vi "Read_data.vi"(0 "DVR in":refnum<data-value>, 5 "Type":string, 11 "error in (no error)":errorcluster) -> (4 "DVR Out":refnum<data-value>, 6 "DATA":T1, 15 "error out":errorcluster)   [LabVIEW 2020, in "With Data.lvclass"]
doc: "Read data to notifier."
uses:
  Classes/Children/Intra-Application/Children/With Data/With Data.lvclass
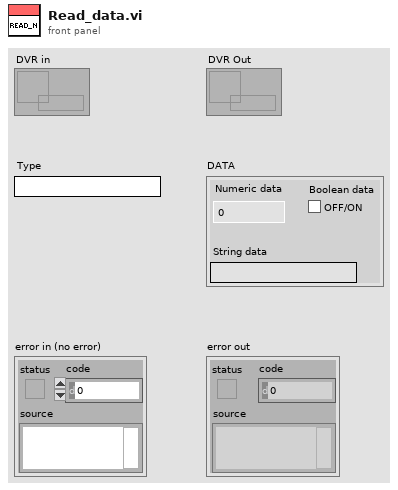
[diagram p1: front panel]
types:
  T1 = cluster{"Numeric data":dbl, "String data":string, "Boolean data":bool}
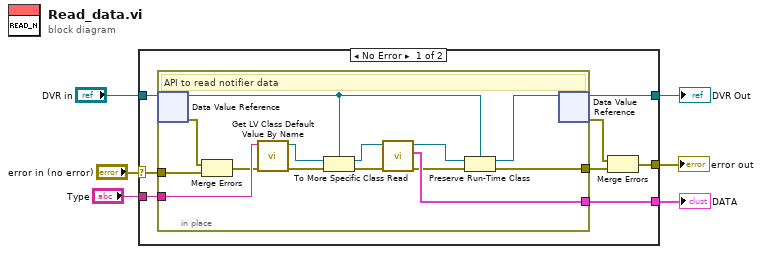
[diagram p0: block diagram]
diagram:
  n1 = case shown="No Error" "error in (no error)" {
    selector: "error in (no error)" -> [w14 w30]
    tunnel: [w11 w30] -> w5
    tunnel: [w10 _] -> w4
    tunnel: "DVR in" -> [w9 w29]
    tunnel: [w8 w29] -> w1
    tunnel: "Type" -> [w7 _]
    frame No Error {
      n2 = in-place "In Place Element Structure" {
        in-place-border: [w18] -> w13
        in-place-border: w14 -> [w27]
        in-place-border: [w20] -> w10
        in-place-border: w7 -> [w22]
        # "API to read notifier data"
        n3 = in-place-dvr #1(w9) -> (w16:refnum<class "With Data.lvclass">, w28:errorcluster)
        n4 = Merge Errors(w28, w27) -> (w21:errorcluster)
        n5 = call <vilib>:"Get LV Class Default Value By Name.vi"("error in (no error)"=w21, "class name"=w22) -> ("error out"=w23:errorcluster, "object"=w25:refnum<class>)  [unwired: 8 in]
        n6 = To More Specific Class(target class=w16, reference=w25, error in=w23) -> (specific class reference=w26:refnum<class "With Data.lvclass">, error out=w24:errorcluster)
        n7 = call-dynamic "Read.vi"("error in (no error)"=w24, "With Data in"=w26) -> ("error out"=w19:errorcluster, "DATA"=w20:T1, "With Data out"=w17:refnum<class "With Data.lvclass">)  [unwired: 7 in]
        n8 = Preserve Run-Time Class(object in=w17, error in=w19, 2:w16) -> (object out=w15:refnum<class "With Data.lvclass">, error out=w18:errorcluster)
        n9 = in-place-dvr #1(w15) -> (w8:refnum<data-value>, w12:errorcluster)
      }
      n10 = Merge Errors(w12, w13) -> (w11:errorcluster)
    }
    frame Error {
    }
  }
  "error out" <- w5
  "DATA" <- w4
  "DVR Out" <- w1
